vi "RunCL - Set Version Info.vi"(11 "Cmd Line Args":string[](array[string])) -> (2 "Error Info":string, 3 "Error Code":i32)   [LabVIEW 2023]
uses:
  <vilib>/AppBuilder/AB_API_Simple/Build Specification Version.ctl
  <vilib>/AppBuilder/AB_API_Simple/Set Build Specification Version (path).vi
  <vilib>/AppBuilder/AB_API_Simple/NI_App_Builder_API.lvlib
panel:
  out "error out":errorcluster
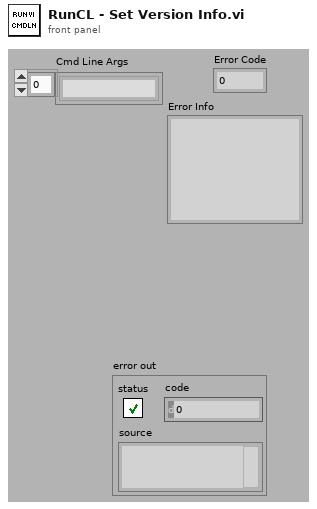
[diagram p1: front panel]
types:
  T1 = typedef "NI_App_Builder_API.lvlib/Build Specification Version.ctl" = cluster{"Major":u16, "Minor":u16, "Fix":u16, "Build":u16}
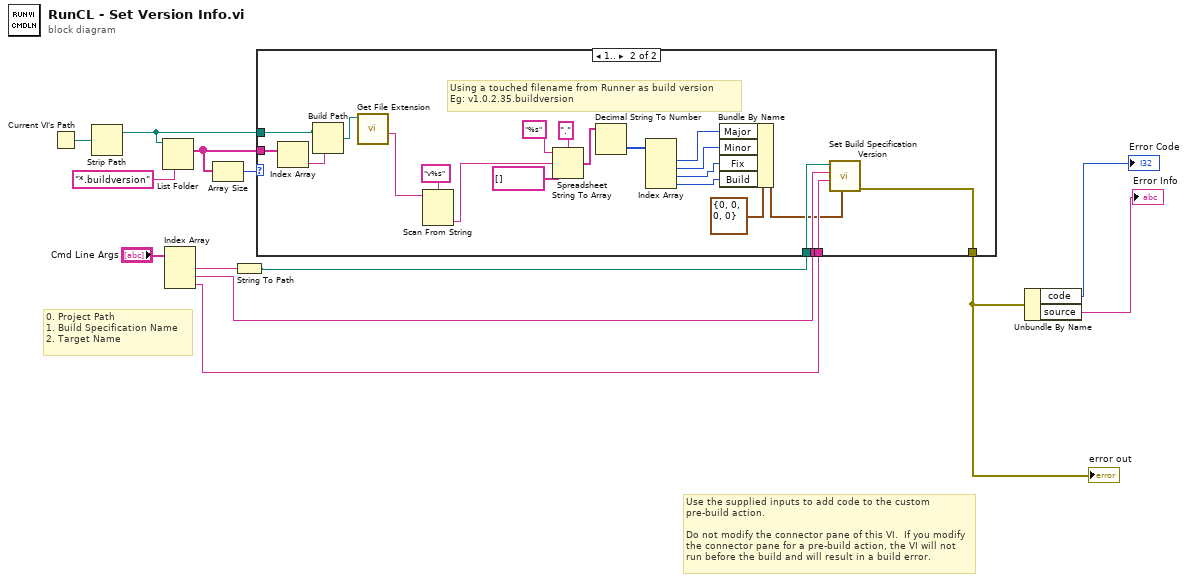
[diagram p0: block diagram]
diagram:
  # "0. Project Path\n1. Build Specification Name\n2. Target Name"
  # "Use the supplied inputs to add code to the custom pre-build action.\n\nDo not modify the connector pane of this VI.  If you modify the connector pane for a pre-build action, the VI will not run before the build and will result in a build error."
  n1 = Current VI's Path() -> (path=w13:path)
  n2 = Strip Path(path=w13) -> (stripped path=w11:path)  [unwired: 1 out]
  n3 = List Folder(path=w11, pattern="*.buildversion") -> (filenames=w10:string[])  [unwired: 2 in, 3 out]
  n4 = Index Array(array="Cmd Line Args") -> (element #1=w7:string, element #2=w5:string, element #3=w4:string)  [unwired: 3 in]
  n5 = Array Size(array=w10) -> (size(s)=w9:i32)
  n6 = String To Path(string=w7) -> (path=w6:path)
  n7 = case shown="1.." w9 {
    tunnel: [_ w14] -> w3
    tunnel: w5 -> [_ w35]
    tunnel: w6 -> [_ w34]
    tunnel: w4 -> [_ w33]
    tunnel: w10 -> [_ w32]
    tunnel: w11 -> [_ w17]
    frame 0, Default {
    }
    frame 1.. {
      # "Using a touched filename from Runner as build version\nEg: v1.0.2.35.buildversion"
      n8 = Index Array(array=w32) -> (element=w16:string)  [unwired: 1 in]
      n9 = Build Path(base path=w17, name or relative path=w16) -> (appended path=w18:path)
      n10 = call <vilib>:"Get File Extension.vi"("file"=w18) -> ("filename without extension"=w15:string)  [unwired: 6 in, 4 out]
      n11 = Scan From String(format string="v%s", input string=w15) -> (output 1=w19:string)  [unwired: 3 in, 3 out]
      n12 = Spreadsheet String To Array(delimiter (Tab)=".", format string="%s", spreadsheet string=w19, array type (2D Dbl)=string[] []) -> (array=w26:string[])
      n13 = Decimal String To Number(string=w26) -> (number=w25:i32[])  [unwired: 2 in, 1 out]
      n14 = Index Array(array=w25) -> (element #1=w24:i32, element #2=w23:i32, element #3=w22:i32, element #4=w21:i32)  [unwired: 4 in]
      n15 = Bundle By Name(cluster=T1 {"Major"=0, "Minor"=0, "Fix"=0, "Build"=0} ("Build Specification Version"), "Major"=w24, "Minor"=w23, "Fix"=w22, "Build"=w21) -> (w27:T1)
      n16 = call-poly <vilib>:"Set Build Specification Version.vi"("Build Specification Version"=w27, "Name of target (My Computer)"=w33, "Name of build specification"=w35, "Path to project"=w34) -> ("error out"=w14:errorcluster)  [unwired: 7 in]
    }
  }
  "error out" <- w3
  n17 = Unbundle By Name(w3) -> ("code"=→"Error Code":i32, "source"=→"Error Info":string)
